vi "Get Entry - Directory.vi"(7 "Directory":string[](array[string]), 8 "error in (no error)":errorcluster, 10 "Key":string, 11 "Registry in":refnum<class "Registry.lvclass">) -> (0 "error out":errorcluster, 1 "Value":variant, 2 "Key Out":string, 4 "Found?":bool)   [LabVIEW 2020, in "BCI-1553 API.lvlib" / "Registry.lvlib" / "Registry.lvclass"]
doc: "Retrieves a Key/Value pair nested in a hierarchy of Registries. The final key in the directory array should be the the Registry that contains the Key/Value pair you want to retrieve."
uses:
  Registry.lvclass
  Registry.lvclass/Registry.ctl
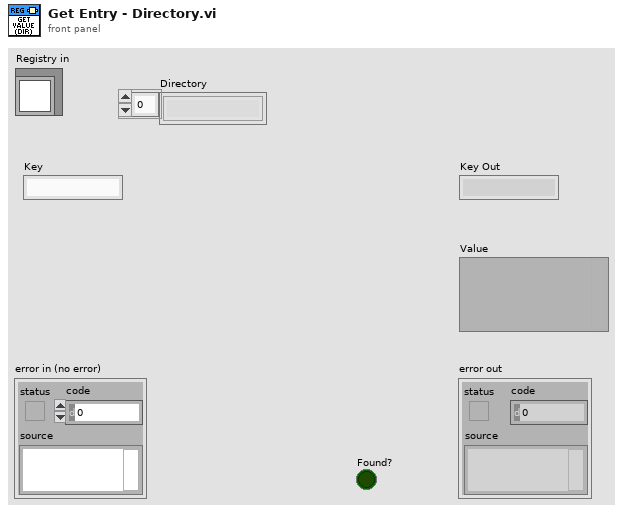
[diagram p1: front panel]
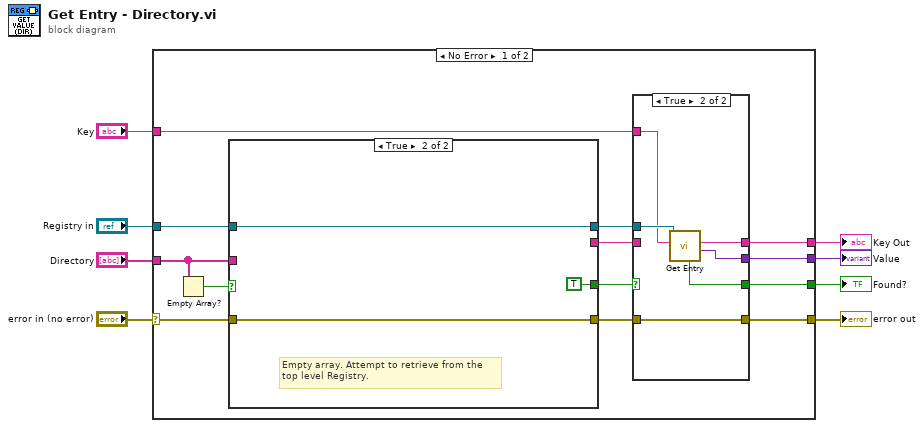
[diagram p0: block diagram]
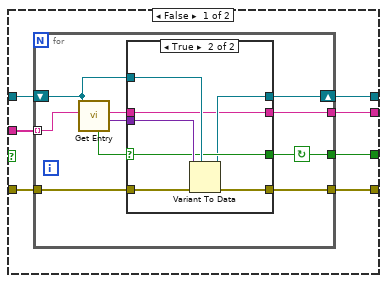
[diagram p2: hidden frame]
diagram:
  n1 = case shown="No Error" "error in (no error)" {
    selector: "error in (no error)" -> [w20 w61]
    tunnel: [w19 w61] -> w7
    tunnel: "Registry in" -> [w21 _]
    tunnel: "Directory" -> [w10 _]
    tunnel: [w12 _] -> w3
    tunnel: [w16 _] -> w4
    tunnel: "Key" -> [w13 _]
    tunnel: [w11 _] -> w1
    frame No Error {
      n2 = Empty Array?(array=w10) -> (empty?=w9:bool)
      n3 = case shown="True" w9 {
        tunnel: w21 -> [w28 w51]
        tunnel: w20 -> [w27 w49]
        tunnel: [w26 w49] -> w18
        tunnel: [w25 TRUE] -> w17
        tunnel: [w24 _] -> w15
        tunnel: [w23 w51] -> w14
        tunnel: w10 -> [w22 _]
        frame False {
          n4 = for {
            tunnel: w22 -> [w38] mode=indexing
            shift-right: [w33] -> w23
            shift-left: w28 -> [w34]
            tunnel: w27 -> [w32]
            tunnel: [w31] -> w26
            tunnel: [w30] -> w24
            tunnel: [w29] -> w25
            stop <- w29 continue-if-true
            n5 = call "Get Entry.vi"("Key"=w38, "Registry in"=w34) -> ("Value"=w37:variant, "Key Out"=w35:string, "Found?"=w36:bool)  [unwired: 6 in, 1 out]
            n6 = case shown="True" w36 {
              selector: w36 -> [w41 w46]
              tunnel: w34 -> [_ w48]
              tunnel: w37 -> [_ w47]
              tunnel: [w41 w46] -> w29
              tunnel: [_ w45] -> w33
              tunnel: w32 -> [w39 w44]
              tunnel: [w39 w43] -> w31
              tunnel: w35 -> [w40 w42]
              tunnel: [w40 w42] -> w30
              frame False {
              }
              frame True {
                n7 = Variant To Data(error in=w44, type=w48, Variant=w47) -> (data=w45:refnum<class "Registry.lvclass">, error out=w43:errorcluster)
              }
            }
          }
        }
        frame True {
          # "Empty array. Attempt to retrieve from the\ntop level Registry."
        }
      }
      n8 = case shown="True" w17 {
        selector: w17 -> [w53 _]
        tunnel: [w52 w60] -> w19
        tunnel: w18 -> [w52 w60]
        tunnel: [w54 w58] -> w16
        tunnel: w15 -> [w54 _]
        tunnel: w14 -> [_ w59]
        tunnel: w13 -> [_ w55]
        tunnel: [w53 w57] -> w12
        tunnel: [_ w56] -> w11
        frame False {
        }
        frame True {
          n9 = call "Get Entry.vi"("Key"=w55, "Registry in"=w59) -> ("Value"=w56:variant, "Key Out"=w58:string, "Found?"=w57:bool)  [unwired: 6 in, 1 out]
        }
      }
    }
    frame Error {
    }
  }
  "error out" <- w7
  "Key Out" <- w4
  "Value" <- w1
  "Found?" <- w3
